vi "All_Off_Relays.vi"() -> ()   [LabVIEW 2023]
uses:
  <vilib>/ULx/Create Channel.llb/ULx Create Channel (DO-Digital Output).vi
  <vilib>/ULx/Write.llb/ULx Write (Digital 1D Bool 1Chan 1Samp).vi
panel:
  out "error out":errorcluster
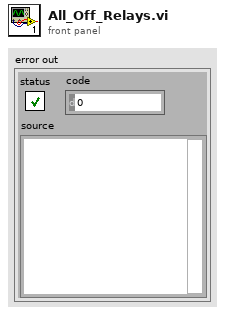
[diagram p1: front panel]
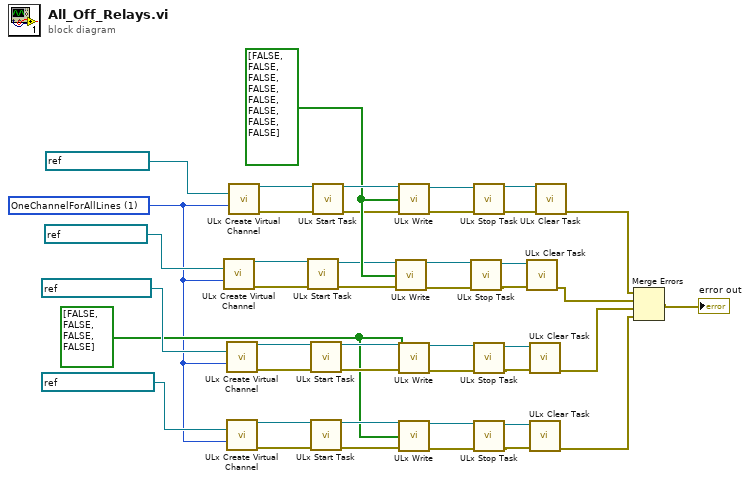
[diagram p0: block diagram]
diagram:
  w7 = 1 items=["OneChannelForEachLine", "OneChannelForAllLines"] ("line grouping")
  w8 = bool[] [FALSE, FALSE, FALSE, FALSE] ("data")
  w38 = bool[] [FALSE, FALSE, FALSE, FALSE, FALSE, FALSE, FALSE, FALSE] ("data")
  n1 = call-poly <vilib>:"ULx Create Virtual Channel.vi"("lines"=refnum<k21> "Dev0/1stPortB", "line grouping"=w7) -> ("task out"=w31:refnum<k24>, "error out"=w30:errorcluster)  [unwired: 12 in]
  n2 = call-poly <vilib>:"ULx Create Virtual Channel.vi"("lines"=refnum<k21> "Dev0/1stPortCL", "line grouping"=w7) -> ("task out"=w23:refnum<k24>, "error out"=w22:errorcluster)  [unwired: 12 in]
  n3 = call-poly <vilib>:"ULx Create Virtual Channel.vi"("lines"=refnum<k21> "Dev0/1stPortCH", "line grouping"=w7) -> ("task out"=w13:refnum<k24>, "error out"=w12:errorcluster)  [unwired: 12 in]
  n4 = call-poly <vilib>:"ULx Create Virtual Channel.vi"("lines"=refnum<k21> "Dev0/1stPortA", "line grouping"=w7) -> ("task out"=w43:refnum<k24>, "error out"=w44:errorcluster)  [unwired: 12 in]
  n5 = call <vilib>:"ULx Start Task.vi"("task in"=w31, "error in"=w30) -> ("task out"=w6:refnum<k24>, "error out"=w29:errorcluster)  [unwired: 12 in]
  n6 = call <vilib>:"ULx Start Task.vi"("task in"=w23, "error in"=w22) -> ("task out"=w20:refnum<k24>, "error out"=w21:errorcluster)  [unwired: 12 in]
  n7 = call <vilib>:"ULx Start Task.vi"("task in"=w13, "error in"=w12) -> ("task out"=w10:refnum<k24>, "error out"=w11:errorcluster)  [unwired: 12 in]
  n8 = call <vilib>:"ULx Start Task.vi"("task in"=w43, "error in"=w44) -> ("task out"=w42:refnum<k24>, "error out"=w37:errorcluster)  [unwired: 12 in]
  n9 = call-poly <vilib>:"ULx Write.vi"("task in"=w6, "data"=w38, "error in"=w29) -> ("task out"=w35:refnum<k24>, "error out"=w34:errorcluster)  [unwired: 10 in, 1 out]
  n10 = call-poly <vilib>:"ULx Write.vi"("task in"=w42, "data"=w38, "error in"=w37) -> ("task out"=w19:refnum<k24>, "error out"=w40:errorcluster)  [unwired: 10 in, 1 out]
  n11 = call-poly <vilib>:"ULx Write.vi"("task in"=w20, "data"=w8, "error in"=w21) -> ("task out"=w27:refnum<k24>, "error out"=w26:errorcluster)  [unwired: 10 in, 1 out]
  n12 = call-poly <vilib>:"ULx Write.vi"("task in"=w10, "data"=w8, "error in"=w11) -> ("task out"=w17:refnum<k24>, "error out"=w16:errorcluster)  [unwired: 10 in, 1 out]
  n13 = call <vilib>:"ULx Stop Task.vi"("error in"=w34, "task in"=w35) -> ("error out"=w32:errorcluster, "task out"=w33:refnum<k24>)  [unwired: 8 in]
  n14 = call <vilib>:"ULx Stop Task.vi"("error in"=w40, "task in"=w19) -> ("error out"=w41:errorcluster, "task out"=w18:refnum<k24>)  [unwired: 8 in]
  n15 = call <vilib>:"ULx Stop Task.vi"("error in"=w26, "task in"=w27) -> ("error out"=w24:errorcluster, "task out"=w25:refnum<k24>)  [unwired: 8 in]
  n16 = call <vilib>:"ULx Stop Task.vi"("error in"=w16, "task in"=w17) -> ("error out"=w14:errorcluster, "task out"=w15:refnum<k24>)  [unwired: 8 in]
  n17 = call <vilib>:"ULx Clear Task.vi"("task in"=w33, "error in"=w32) -> ("error out"=w3:errorcluster)  [unwired: 13 in]
  n18 = call <vilib>:"ULx Clear Task.vi"("task in"=w25, "error in"=w24) -> ("error out"=w2:errorcluster)  [unwired: 13 in]
  n19 = call <vilib>:"ULx Clear Task.vi"("task in"=w15, "error in"=w14) -> ("error out"=w1:errorcluster)  [unwired: 13 in]
  n20 = call <vilib>:"ULx Clear Task.vi"("task in"=w18, "error in"=w41) -> ("error out"=w4:errorcluster)  [unwired: 13 in]
  n21 = Merge Errors(w4, w3, w2, w1) -> (→"error out":errorcluster)
